vi "Sensor State.vi"(8 "error in (no error)":errorcluster, 11 "VISA resource name":refnum<visa-resource-name>) -> (0 "error out":errorcluster, 2 "State Data":T1, 3 "VISA resource name out":refnum<visa-resource-name>)   [LabVIEW 2014, in "Hokuyo URG Series.lvlib"]
doc: "Returns the current state of the sensor in a cluster data type. The data returned may need to be manipulated using string functions. Refer to the instrument manual for information on the format of the returned data."
uses:
  Hokuyo URG Series.lvlib
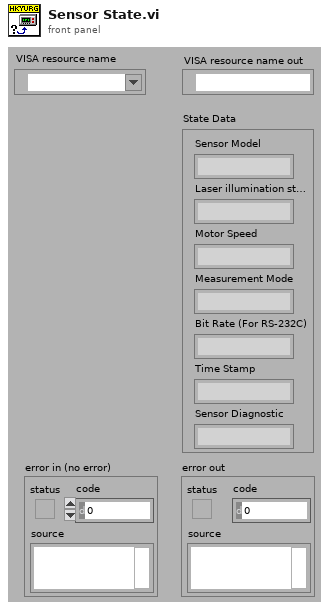
[diagram p1: front panel]
types:
  T1 = cluster{"Sensor Model":string, "Laser illumination state":string, "Motor Speed":string, "Measurement Mode":string, "Bit Rate (For RS-232C)":string, "Time Stamp":string, "Sensor Diagnostic":string}
  T2 = cluster{"[0]":string, "[1]":string, "[2]":string, "[3]":string, "[4]":string, "[5]":string, "[6]":string}
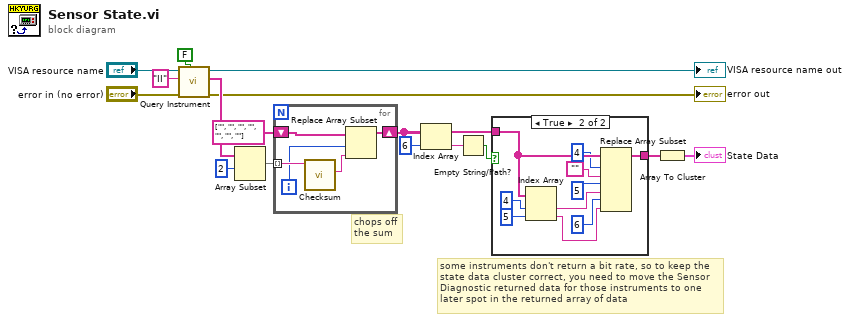
[diagram p0: block diagram]
diagram:
  # "chops off the sum"
  # "some instruments don't return a bit rate, so to keep the state data cluster correct, you need to move the Sensor Diagnostic returned data for those instruments to one later spot in the returned array of data"
  n1 = call "Query Instrument.vi"("Error Query (Enabled)"=FALSE, "error in"="error in (no error)", "Command"="II", "VISA Resource Name"="VISA resource name") -> ("error out"=→"error out":errorcluster, "Response Strings"=w11:string[], "VISA Resource Name Out"=→"VISA resource name out":refnum<visa-resource-name>)  [unwired: 5 in]
  n2 = Array Subset(array=w11, index=2) -> (w7:string[])  [unwired: 1 in]
  n3 = for {
    tunnel: w7 -> [w21] mode=indexing
    shift-right: [w19] -> w3
    shift-left: string[] ["", "", "", "", "", "", ""] -> [w20]
    i -> [w17]
    n4 = call "Checksum.vi"("Input"=w21) -> ("Data Buffer"=w18:string)  [unwired: 9 in, 1 out]
    n5 = Replace Array Subset(array=w20, new element=w18, index=w17) -> (w19:string[])
  }
  n6 = Index Array(array=w3, index=6) -> (element=w5:string)
  n7 = Empty String/Path?(string/path=w5) -> (empty?=w4:bool)
  n8 = case shown="True" w4 {
    tunnel: w3 -> [w22 w32]
    tunnel: [w22 w26] -> w2
    frame False {
    }
    frame True {
      n9 = Index Array(array=w32, index #1=4 ("index"), index #2=5 ("index")) -> (element #1=w28:string, element #2=w23:string)
      n10 = Replace Array Subset(array=w32, new element #1="", index #1=4 ("index"), new element #2=w28, index #2=5 ("index"), new element #3=w23, index #3=6 ("index")) -> (w26:string[])
    }
  }
  n11 = Array To Cluster(array=w2) -> (cluster=→"State Data":T2)
